vi "Get Data.vi"(6 "Index in":i32, 8 "error in (no error)":errorcluster, 10 "Data":T1[](array[typedef]), 11 "Composite Object in":refnum<class "CConfig Object.lvclass">) -> (0 "error out":errorcluster, 2 "Data":string[](array[string]), 3 "Composite Object out":refnum<class "CConfig Object.lvclass">)   [LabVIEW 2013, in "CConfig Object.lvclass"]
doc: "Copyright 2018, Carya Automatisering, Wiebe Walstra."
uses:
  CConfig Object.lvclass
  Data.ctl
  CConfig Object.lvclass/CConfig Object.ctl
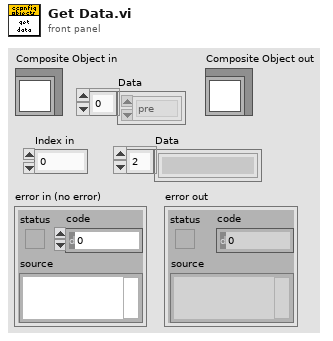
[diagram p1: front panel]
types:
  T1 = typedef "CConfig Object.lvclass/Data.ctl" = enum16{"pre", "name", "middle", "value", "post", "newline", "persistant", "tagged", "type"}
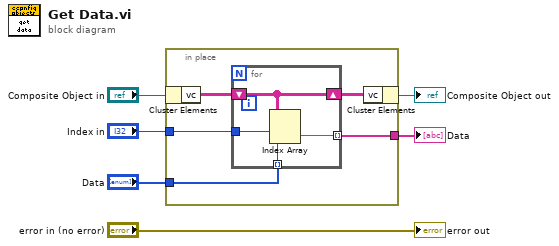
[diagram p0: block diagram]
diagram:
  n1 = in-place {
    in-place-border: "Index in" -> [w11]
    in-place-border: [w10] -> w4
    in-place-border: "Data" -> [w8]
    n2 = in-place-cluster #1("Composite Object in") -> ("vc"=w9:string[][])
    n3 = for {
      tunnel: w11 -> [w15]
      tunnel: [w14] -> w10 mode=indexing
      tunnel: w8 -> [w13] mode=indexing
      shift-right: [w12] -> w7
      shift-left: w9 -> [w12]
      n4 = Index Array(array=w12, index (row)=w15, index (col)=w13) -> (element=w14:string)
    }
    n5 = in-place-cluster #1("vc"=w7) -> (→"Composite Object out":refnum<class "CConfig Object.lvclass">)
  }
  "Data" <- w4
  "error out" <- "error in (no error)"
